vi "Stream to TDMS Files (Optimized Performance).vi"() -> ()   [LabVIEW 2020]
doc: "The Stream to TDMS Files (Optimized Performance) example shows how to save images to a TDMS file when using a ring acquisition. The TDMS API has been optimized to take advantage of asynchronous writes, parallel background workers, disk reservation, and disabling buffering to improve write perfromance. Read the comments on the block diagram of this VI to learn more about these optimization options."
uses:
  <vilib>/vision/driver/IMAQdx.llb/IMAQdx Acquisition Mode.ctl
  Program Files (x86)/National Instruments/LabVIEW 2020/examples/Vision Acquisition/NI-IMAQdx/Stream to Disk/SubVIs/TDMS Write Settings.ctl
  <vilib>/vision/Image Controls.llb/IMAQ Image.ctl
  <vilib>/vision/driver/IMAQdx.llb/IMAQdx Buffer Number Mode.ctl
  <vilib>/Utility/High Resolution Relative Seconds.vi
  Program Files (x86)/National Instruments/LabVIEW 2020/examples/Vision Acquisition/NI-IMAQdx/Stream to Disk/SubVIs/TDMS File Initialization (Write).vi
  <vilib>/vision/EDVR.llb/IMAQ ImageToEDVR.vi
  <vilib>/vision/EDVR.llb/IMAQ ImageToEDVR 1D U8.vi
  <vilib>/vision/EDVR.llb/IMAQ ImageToEDVR 1D I16.vi
  <vilib>/vision/EDVR.llb/IMAQ ImageToEDVR 1D U32.vi
  <vilib>/vision/EDVR.llb/IMAQ ImageToEDVR 1D U16.vi
  <vilib>/vision/driver/NI_Vision_Acquisition_Software.lvlib
  <resource>/objmgr/imaqdx.rc
panel:
  out "Optimizations":T1
  in  "Skip Count":u32
  out "Images Saved Per Second":dbl
  out "Images Acquired Per Second":dbl
  in  "Images per TDMS":i64=10000
  out "Write Speed":dbl(graph) caption="Image File Write Speed"
  in  "Destination Folder":path
  out "Images Behind":u32
  in  "Number of Images":i32=30
  in  "Camera Name":refnum<k21> caption="IMAQdx Session"
  in  "Stop":bool
  # "Overview: Demonstrates how to stream images to TDMS files when using a ring acquisition.\nRequirements: Vision Acquisition Software\nInstructions:\n1. Select the Camera Name\n2. Run the VI\n3. Increase the Skip Count if Images Behind is greater than 0."
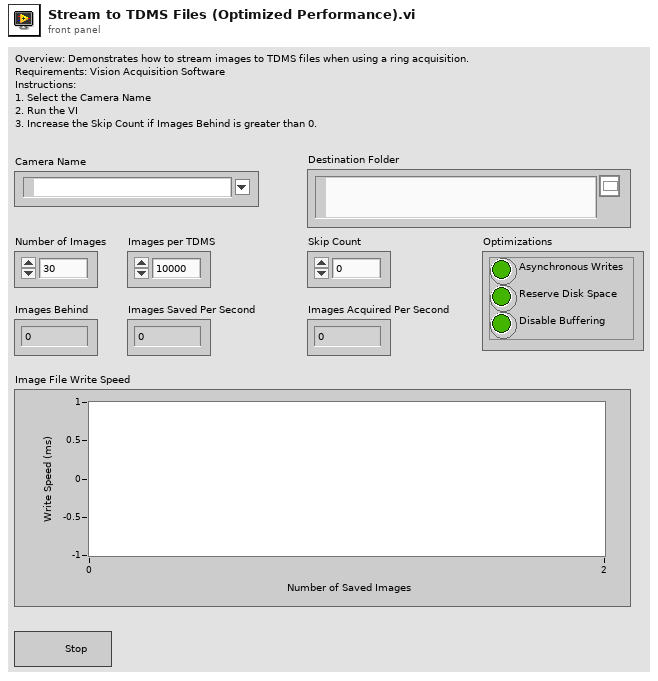
[diagram p1: front panel]
types:
  T1 = cluster{"Asynchronous Writes":bool, "Reserve Disk Space":bool, "Disable Buffering":bool}
  T2 = typedef "TDMS Write Settings.ctl" = cluster{"Asynchronous":bool, "Disable Buffering if Supported":bool, "Reserved Images":i64, "Fail if Reservation Fails":bool}
  T3 = typedef "NI_Vision_Acquisition_Software.lvlib/IMAQdx Acquisition Mode.ctl" = enum32{"One Shot", "Continuous"}
  T4 = typedef "IMAQdx.ctl" = refnum<k21>
  T5 = typedef "IMAQ Image.ctl" = refnum<image>
  T6 = typedef "Image Type" = u32
  T7 = cluster{"Image Type":T6, "Async File Format":bool}
  T8 = cluster{"Asynchronous Write":bool, "Reserve Disk Space":bool, "Disable Buffering":bool}
  T9 = typedef "NI_Vision_Acquisition_Software.lvlib/IMAQdx Buffer Number Mode.ctl" = enum32{"Next", "Last", "Buffer Number", "Every", "Last New"}
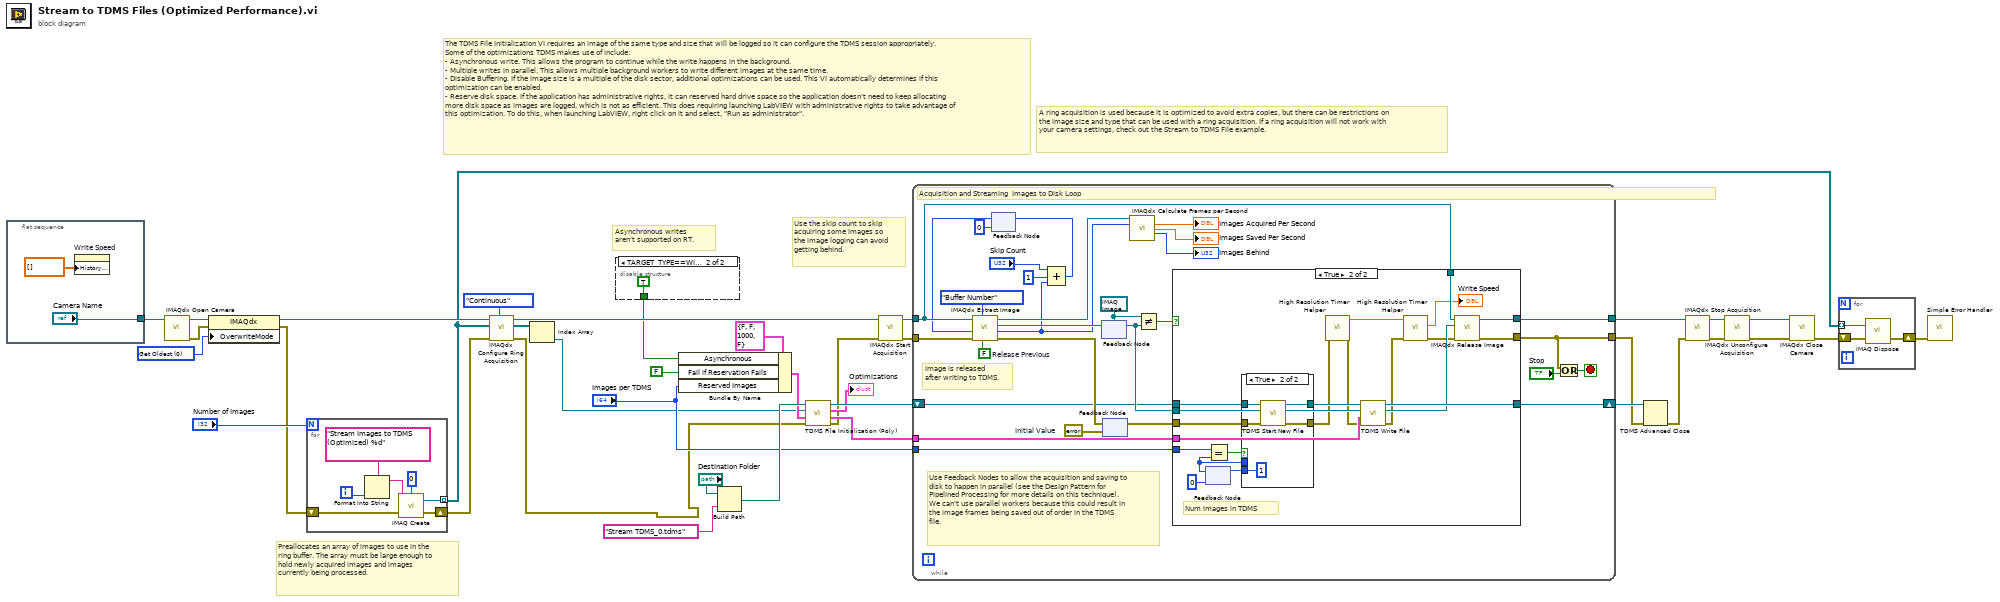
[diagram p0: block diagram]
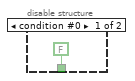
[diagram p2: hidden frame]
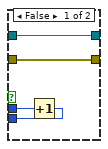
[diagram p4: hidden frame]
diagram:
  w11 = u32 0 items=["Get Oldest"=0, "Fail"=2, "Get Newest"=3] ("OverwriteMode")
  # "The TDMS File Initialization VI requires an image of the same type and size that will be logged so it can configure the TDMS session appropriately. Some of the optimizations TDMS makes use of include:\n- Asynchronous write. This allows the program to continue while the write happens in the background.\n- Multiple writes in parallel. This allows multiple background workers to write different images at the same time.\n- Disable Buffering. If the image size is a multiple of the disk sector, additional optimizations can be used. This VI automatically determines if this optimization can be enabled.\n- Reserve disk space. If the application has administrative rights, it can reserved hard drive space so the application doesn't need to keep allocating more disk space as images are logged, which is not as efficient. This does requiring launching LabVIEW with administrative rights to take advantage of this optimization. To do this, when launching LabVIEW, right click on it and select, \"Run as administrator\"."
  # "Asynchronous writes aren't supported on RT."
  # "Use the skip count to skip acquiring some images so the image logging can avoid getting behind."
  # "A ring acquisition is used because it is optimized to avoid extra copies, but there can be restrictions on the image size and type that can be used with a ring acquisition. If a ring acquisition will not work with your camera settings, check out the Stream to TDMS File example."
  # "Preallocates an array of images to use in the ring buffer. The array must be large enough to hold newly acquired images and images currently being processed."
  n1 = flat-sequence {
    tunnel: ["Camera Name"] -> w38
    frame #0 {
      n2 = property on="Write Speed" class="WFChart (strict)"("History Data"=dbl[] []) -> ()  [unwired: 2 in, 2 out]
    }
  }
  n3 = call <vilib>:"IMAQdx Open Camera.vi"("Session In"=w38) -> ("error out"=w33:errorcluster, "Session Out"=w34:T4)  [unwired: 2 in, 7 out]
  n4 = property class="IMAQdx"(reference=w34, error in=w33, "OverwriteMode"=w11) -> (reference out=w31:T4, error out=w7:errorcluster)
  n5 = for {
    N: "Number of Images" -> [_]
    tunnel: [w46] -> w6 mode=indexing
    shift-right: [w45] -> w5
    shift-left: w7 -> [w47]
    i -> [w44]
    n6 = Format Into String(format string="Stream Images to TDMS (Optimized) %d" ("Image Name"), w44) -> (resulting string=w43:string)  [unwired: 2 in, 1 out]
    n7 = call "IMAQ Create"("Border Size"=0, "Image Name"=w43, "error in (no error)"=w47) -> ("New Image"=w46:T5, "error out"=w45:errorcluster)  [unwired: 1 in, 1 out]
  }
  n8 = call <vilib>:"IMAQdx Configure Ring Acquisition.vi"("Mode"=IMAQdx_Acquisition_Mode."Continuous" ("Continuous?"), "error in"=w5, "Images"=w6, "Session In"=w31) -> ("error out"=w1:errorcluster, "Images Out"=w4:T5[], "Session Out"=w28:T4)  [unwired: 5 in]
  n9 = Index Array(array=w4) -> (element=w3:T5)  [unwired: 1 in]
  n10 = disable-structure shown="TARGET_TYPE==Windows" {
    disable-tunnel: [FALSE ("Asynchronous") TRUE ("Asynchronous")] -> w13
    frame condition #0 {
    }
    frame condition #1 (active) {
    }
  }
  n11 = Bundle By Name(cluster=T2 {"Asynchronous"=FALSE, "Disable Buffering if Supported"=FALSE, "Reserved Images"=1000, "Fail if Reservation Fails"=FALSE} ("Write Settings"), "Asynchronous"=w13, "Fail if Reservation Fails"=FALSE, "Reserved Images"="Images per TDMS") -> (w12:T2)
  n12 = Build Path(base path="Destination Folder", name or relative path="Stream TDMS_0.tdms") -> (appended path=w20:path)
  n13 = call-poly "TDMS File Initialization (Poly).vi"("error in (no error)"=w1, "Write Settings"=w12, "Image In"=w3, "File Path"=w20) -> ("error out"=w2:errorcluster, "Write Settings Out"=w18:T7, "Optimizations Configured"=→"Optimizations":T8, "TDMS Refnum Out"=w21:refnum<k34>)  [unwired: 4 in]
  n14 = call <vilib>:"IMAQdx Start Acquisition.vi"("error in"=w2, "Session In"=w28) -> ("error out"=w24:errorcluster, "Session Out"=w25:T4)  [unwired: 8 out]
  n15 = while {
    tunnel: w24 -> [w78]
    tunnel: w25 -> [w74]
    tunnel: [w75] -> w26
    tunnel: [w63] -> w16
    shift-right: [w76] -> w17
    shift-left: w21 -> [w60]
    tunnel: "Images per TDMS" -> [w59]
    tunnel: w18 -> [w62]
    stop <- w65 stop-if-true
    w50 = errorcluster {"status"=FALSE, "code"=0, "source"=""}  # Initial Value
    w72 = FALSE  # Release Previous
    w68 = T5 refnum ("Image Out")
    # "Use Feedback Nodes to allow the acquisition and saving to disk to happen in parallel (see the Design Pattern for Pipelined Processing for more details on this technique). We can't use parallel workers because this could result in the image frames being saved out of order in the TDMS file."
    # "Image is released after writing to TDMS."
    # "Acquisition and Streaming  Images to Disk Loop"
    n16 = feedback #1(u32 0) -> (w52:u32)
    n17 = call <vilib>:"IMAQdx Extract Image.vi"("Release Previous (true)"=w72, "Buffer Number Mode (Next)"=IMAQdx_Buffer_Number_Mode."Buffer Number" ("Buffer Number Mode"), "error in"=w78, "Buffer Number In"=w52, "Session In"=w74) -> ("error out"=w61:errorcluster, "Buffer Number Out"=w54:u32, "Image Out"=w70:T5, "Session Out"=w71:T4)  [unwired: 3 in]
    n18 = Compound Arithmetic op=ADD("Skip Count", u32 1 ("value"), w54) -> (w55:u32)
    n19 = feedback-in #1(w55) -> ()
    n20 = feedback-in #2(w70) -> ()
    n21 = feedback #2(w68) -> (w66:T5)
    n22 = feedback-in #3(w61) -> ()
    n23 = feedback #3(w50) -> (w69:errorcluster)
    n24 = call <vilib>:"IMAQdx Calculate Frames per Second.vi"("Session In"=w71, "Buffer Number"=w54) -> ("Acquired Frames per Second"=→"Images Acquired Per Second":dbl, "Processed Frames per Second"=→"Images Saved Per Second":dbl, "Images Behind"=→"Images Behind":i32)  [unwired: 7 in, 4 out]
    n25 = Not Equal?(x=w68, y=w66) -> (x != y?=w67:bool)
    n26 = case shown="True" w67 {
      tunnel: w60 -> [w79 w94]
      tunnel: w66 -> [_ w96]
      tunnel: w69 -> [w80 w92]
      tunnel: [w79 w98] -> w76
      tunnel: [w81 w101] -> w75
      tunnel: w74 -> [w81 w100]
      tunnel: [w80 w99] -> w63
      tunnel: w62 -> [_ w97]
      tunnel: w59 -> [_ w90]
      frame False {
        # "First iteration doesn't have valid image for this pipelined stage."
      }
      frame True {
        # "Num Images in TDMS"
        n27 = feedback #4(i64 0) -> (w89:i64)
        n28 = Equal?(x=w90, y=w89) -> (x = y?=w91:bool)
        n29 = case shown="True" w91 {
          tunnel: [w105 i64 1] -> w88
          tunnel: w94 -> [w104 w109]
          tunnel: [w104 w108] -> w93
          tunnel: w92 -> [w103 w106]
          tunnel: [w103 w107] -> w87
          tunnel: w89 -> [w102 _]
          frame False {
            n30 = Increment(x=w102) -> (x+1=w105:i64)
          }
          frame True {
            n31 = call "TDMS Start New File.vi"("error in"=w106, "Previous TDMS Refnum In"=w109) -> ("error out"=w107:errorcluster, "New TDMS Refnum Out"=w108:refnum<k34>)  [unwired: 8 in]
          }
        }
        n32 = feedback-in #4(w88) -> ()
        n33 = call "High Resolution Timer Helper.vi"("error in (no error)"=w87) -> ("error out"=w86:errorcluster, "Current Time"=w84:dbl)  [unwired: 8 in, 1 out]
        n34 = call "TDMS Write File.vi"("error in"=w86, "Write Settings"=w97, "Image"=w96, "TDMS Ref In"=w93) -> ("error out"=w85:errorcluster, "TDMS Ref Out"=w98:refnum<k34>)  [unwired: 6 in]
        n35 = call "High Resolution Timer Helper.vi"("error in (no error)"=w85, "Previous Time"=w84) -> ("error out"=w83:errorcluster, "Time Difference (ms)"=→"Write Speed":dbl)  [unwired: 7 in, 1 out]
        n36 = call <vilib>:"IMAQdx Release Image.vi"("error in"=w83, "Image"=w96, "Session In"=w100) -> ("error out"=w99:errorcluster, "Session Out"=w101:T4)  [unwired: 7 in]
      }
    }
    n37 = Or(x=w63, y="Stop") -> (x .or. y?=w65:bool)
  }
  n38 = TDMS Advanced Close(8:w16, 11:w17) -> (0:w15:errorcluster)  [unwired: 2 in, 1 out]
  n39 = call <vilib>:"IMAQdx Stop Acquisition.vi"("error in"=w15, "Session In"=w26) -> ("error out"=w29:errorcluster, "Session Out"=w30:T4)  [unwired: 8 out]
  n40 = call <vilib>:"IMAQdx Unconfigure Acquisition.vi"("error in"=w29, "Session In"=w30) -> ("error out"=w37:errorcluster, "Session Out"=w36:T4)  [unwired: 8 out]
  n41 = call <vilib>:"IMAQdx Close Camera.vi"("error in"=w37, "Session In"=w36) -> ("error out"=w32:errorcluster)  [unwired: 9 out]
  n42 = for {
    shift-right: [w112] -> w8
    shift-left: w32 -> [w113]
    tunnel: w6 -> [w111] mode=indexing
    n43 = call "IMAQ Dispose"("Image"=w111, "error in (no error)"=w113) -> ("error out"=w112:errorcluster)  [unwired: 4 in]
  }
  n44 = call <vilib>:"Simple Error Handler.vi"("error in (no error)"=w8) -> ()  [unwired: 4 in, 5 out]
